vi "can开关切换.vi"(0 "输入切换ID":u8, 1 "输出切换ID":u8, 3 "函数类型":i32) -> (9 "成功？":bool)   [LabVIEW 2010]
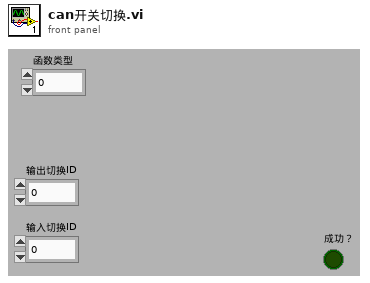
[diagram p1: front panel]
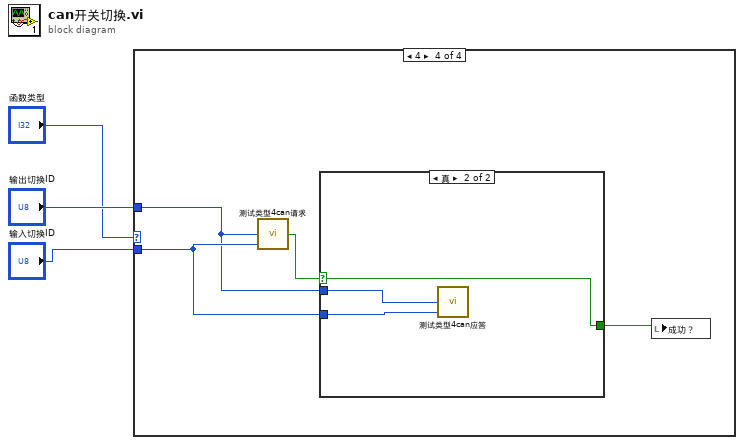
[diagram p0: block diagram]
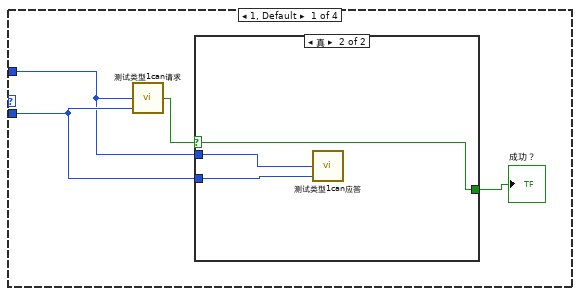
[diagram p2: hidden frame]
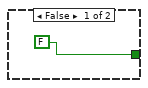
[diagram p3: hidden frame]
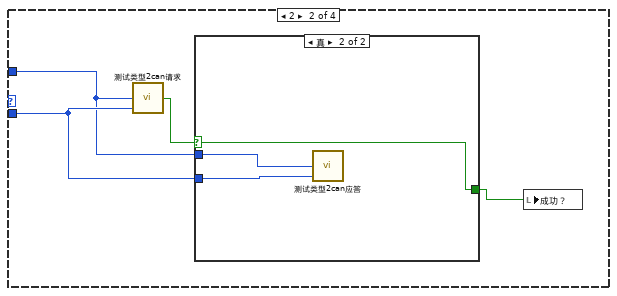
[diagram p4: hidden frame]
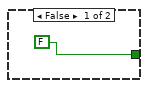
[diagram p5: hidden frame]
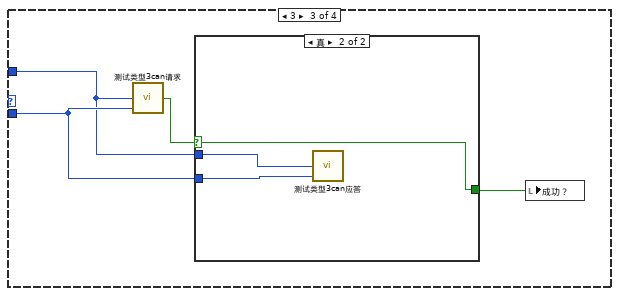
[diagram p6: hidden frame]
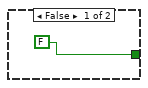
[diagram p7: hidden frame]
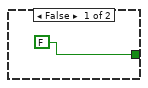
[diagram p8: hidden frame]
diagram:
  n1 = case shown="4" "函数类型" {
    tunnel: "输入切换ID" -> [w6 w15 w23 w31]
    tunnel: "输出切换ID" -> [w4 w13 w21 w29]
    frame 1, Default {
      n2 = call "测试类型1can请求.vi"("输入切换ID"=w6, "输出切换ID"=w4) -> ("发送成功?"=w5:bool)  [unwired: 3 in]
      n3 = case shown="真" w5 {
        selector: w5 -> [_ w9]
        tunnel: [FALSE w9] -> w7
        tunnel: w4 -> [_ w11]
        tunnel: w6 -> [_ w10]
        frame False {
        }
        frame True {
          n4 = call "测试类型1can应答.vi"("输出切换ID"=w11, "输入切换ID"=w10) -> ()  [unwired: 6 in, 1 out]
        }
      }
      "成功？" <- w7
    }
    frame 2 {
      n5 = call "测试类型2can请求.vi"("输入切换ID"=w15, "输出切换ID"=w13) -> ("发送成功?"=w14:bool)  [unwired: 3 in]
      n6 = case shown="真" w14 {
        selector: w14 -> [_ w17]
        tunnel: [FALSE w17] -> w12
        tunnel: w13 -> [_ w19]
        tunnel: w15 -> [_ w18]
        frame False {
        }
        frame True {
          n7 = call "测试类型2can应答.vi"("输出切换ID"=w19, "输入切换ID"=w18) -> ()  [unwired: 6 in, 1 out]
        }
      }
      n8 = local write "成功？"(w12) -> ()
    }
    frame 3 {
      n9 = call "测试类型3can请求.vi"("输入切换ID"=w23, "输出切换ID"=w21) -> ("发送成功?"=w22:bool)  [unwired: 3 in]
      n10 = case shown="真" w22 {
        selector: w22 -> [_ w25]
        tunnel: [FALSE w25] -> w20
        tunnel: w21 -> [_ w27]
        tunnel: w23 -> [_ w26]
        frame False {
        }
        frame True {
          n11 = call "测试类型3can应答.vi"("输出切换ID"=w27, "输入切换ID"=w26) -> ()  [unwired: 6 in, 1 out]
        }
      }
      n12 = local write "成功？"(w20) -> ()
    }
    frame 4 {
      n13 = call "测试类型4can请求.vi"("输入切换ID"=w31, "输出切换ID"=w29) -> ("发送成功?"=w30:bool)  [unwired: 3 in]
      n14 = case shown="真" w30 {
        selector: w30 -> [_ w33]
        tunnel: [FALSE w33] -> w28
        tunnel: w29 -> [_ w35]
        tunnel: w31 -> [_ w34]
        frame False {
        }
        frame True {
          n15 = call "测试类型4can应答.vi"("输出切换ID"=w35, "输入切换ID"=w34) -> ()  [unwired: 6 in, 1 out]
        }
      }
      n16 = local write "成功？"(w28) -> ()
    }
  }
